vi "ReadCtlsFromFile.vi"(10 "ControlsToLoad":refnum<vi>[](array[refnum]), 11 "selected path":path) -> (0 "error out":errorcluster)   [LabVIEW 2015]
uses:
  <vilib>/NI/GXML/GXML.lvlib
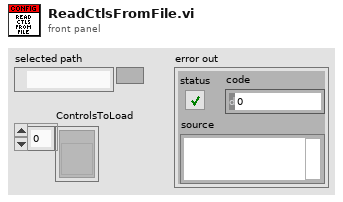
[diagram p1: front panel]
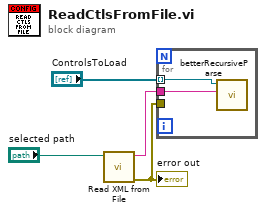
[diagram p0: block diagram]
diagram:
  n1 = call <vilib>:"Read XML from File.vi"("XML File Path"="selected path") -> ("error out"=w4:errorcluster, "XML String Out"=w2:string)  [unwired: 9 in]
  "error out" <- w4
  n2 = for {
    tunnel: w2 -> [w5]
    tunnel: "ControlsToLoad" -> [w6] mode=indexing
    tunnel: w4 -> [_]
    n3 = call "betterRecursiveParse.vi"("XML String in"=w5, "Control in"=w6) -> ()  [unwired: 10 in]
  }
